vi "Get Measurements P1.vi"(0 "Image In":T1, 11 "Error In":errorcluster) -> (1 "Outer Ring":sgl format="%.2f", 2 "Top Outer":sgl format="%.2f", 3 "Top Inner":sgl format="%.2f", 4 "Image Out":T1, 13 "Number of Matches (Locate P1)":i32, 15 "Error Out":errorcluster)   [LabVIEW 2020]
uses:
  <vilib>/vision/Image Controls.llb/IMAQ Image.ctl
  <vilib>/vision/Pattern Matching.llb/IMAQ Curve Parameters.ctl
  <vilib>/vision/Pattern Matching.llb/IMAQ Match Range Setting.ctl
  <vilib>/vision/Pattern Matching.llb/IMAQ Geometric Pattern 2 Advanced Match Options.ctl
  <vilib>/vision/Image Controls.llb/Vision Info Type2.ctl
  <vilib>/vision/Measure.llb/Edge Options.ctl
  <vilib>/vision/Measure.llb/Edge Polarity.ctl
  <vilib>/vision/NI_Vision_Development_Module.lvlib
panel:
  in  "Template File Path":path=path "C:/Users/serce/Desktop/Smart Vision System Testbench/P1 Pattern.png"
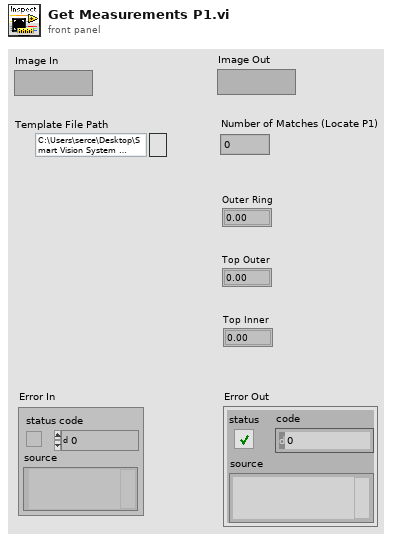
[diagram p1: front panel]
types:
  T1 = typedef "IMAQ Image.ctl" = refnum<image>
  T2 = cluster{"Contrast":i32, "Filter width":i32, "Steepness":i32, "Subsampling Ratio":u32, "Show Search Area":bool, "Show Search Lines":bool, "Show Edges Found":bool, "Show Result":bool}
  T3 = cluster{"Global Rectangle":i32[], "Contours":cluster{"ID":enum32{"External", "Internal"}, "Type":u32, "Coordinates":i32[]}[]}
  T4 = cluster{"Origin":cluster{"X":sgl, "Y":sgl}, "Angle (deg)":sgl, "Axis Reference":u32}
  T5 = enum16{"Reset", "Update Coordinate System", "Get Coordinate System"}
  T6 = typedef "Edge Options.ctl" = cluster{"Edge Polarity":T7, "Kernel Size":u32, "Width":u32, "Minimum Edge Strength":sgl, "Interpolation Type":enum32{"Zero Order", "Bilinear", "Quadratic", "Cubic", "Bilinear Fixed"}, "Data Processing Method":enum32{"Average", "Median"}}
  T7 = typedef "Edge Polarity.ctl" = u32
  T8 = cluster{"Search  Direction":u32, "Edge Options":T6, "Show Search Area":bool, "Show Search Lines":bool, "Show Edges Found":bool, "Show Result":bool, "Search Area Color":u32, "Search Lines Color":u32, "Edge Locations Color":u32, "Result Color":u32, "Overlay Group Name":string}
  T9 = cluster{"Process":enum16{"Get First Edge", "Get First + Last Edge", "Get All Edges", "Get Best Edge"}, "Step Size":i32, "Max Pixel Radius":i32}
  T10 = cluster{"Origin Pixel":cluster{"X":sgl, "Y":sgl}, "Angle Relative to Horizontal (deg)":sgl, "Axis Reference":u32}
  T11 = typedef "Vision Info Type2.ctl" = u32
  T12 = typedef "Simple Grid Descriptor" = cluster{"X Step":sgl, "Y Step":sgl, "Unit":T13}
  T13 = typedef "Image Unit" = enum32{"Undefined", "Angström", "Micrometer", "Millimeter", "Centimeter", "Meter", "Kilometer", "Microinch", "Inch", "Feet", "Nautical miles", "Standard miles", "Steps"}
  T14 = enum16{"Horizontal Motion", "Vertical Motion", "Horizontal and Vertical Motion", "Horizontal, Vertical and Angular Motion"}
  T15 = typedef "IMAQ Curve Parameters.ctl" = cluster{"Extraction Mode":u32, "Edge Threshold":i32, "Edge Filter Size":u32, "Min Length":i32, "Row Search Step Size":i32, "Col Search Step Size":i32, "Max Endpoint Gap":i32, "Closed":bool, "Subpixel":bool}
  T16 = typedef "IMAQ Match Range Setting.ctl" = cluster{"Match Constraints":u32, "Min":dbl, "Max":dbl}
  T17 = typedef "IMAQ Geometric Pattern 2 Advanced Match Options.ctl" = u16
  T18 = cluster{"Curve Parameters":T15, "Match Mode":cluster{"Rotation":bool, "Scale":bool, "Occlusion":bool, "Reserved 1":bool, "Reserved 2":bool, "Reserved 3":bool}, "Range Settings":T16[], "Number of Matches":i32, "Minimum Match Score":sgl, "SubPixel Accuracy":bool, "Adv. Geometric Match Options 2":cluster{"Setup Data Item":T17, "Item Value":dbl}[]}
  T19 = typedef "IMAQ GM Match Report.ctl" = cluster{"Position":cluster{"x":sgl, "y":sgl}, "Angle":sgl, "Scale":sgl, "Score":sgl, "Bounding Box":cluster{"x":sgl, "y":sgl}[], "Contrast Reversed":bool, "Occlusion %":sgl, "Template Target Curve Score":sgl, "Target Template Curve Score":sgl, "Correlation Score":sgl}
  T20 = cluster{"Origin Pixel":cluster{"X":sgl, "Y":sgl}, sgl, "Axis Reference":u32}
  T21 = typedef "IMAQ Coordinate System" = cluster{"Reference System":cluster{"Origin":cluster{"X":sgl, "Y":sgl}, "Angle (deg)":sgl, "Axis Reference":u32}, "Measurement System":cluster{"Origin":cluster{"X":sgl, "Y":sgl}, "Angle (deg)":sgl, "Axis Reference":u32}}
  T22 = typedef "ROI Descriptor" = cluster{"Global Rectangle":i32[], "Contours":cluster{"ID":enum32{"External", "Internal"}, "Type":u32, "Coordinates":i32[]}[]}
  T23 = cluster{"Center (Pixels)":cluster{"X":sgl, "Y":sgl}, "Radius (Pixels)":dbl, "Center (Real-World)":cluster{"X":sgl, "Y":sgl}, "Radius (Real-World)":dbl, "Roundness (Real-World)":dbl, "Average Strength":dbl, "Average SNR (dB)":dbl}
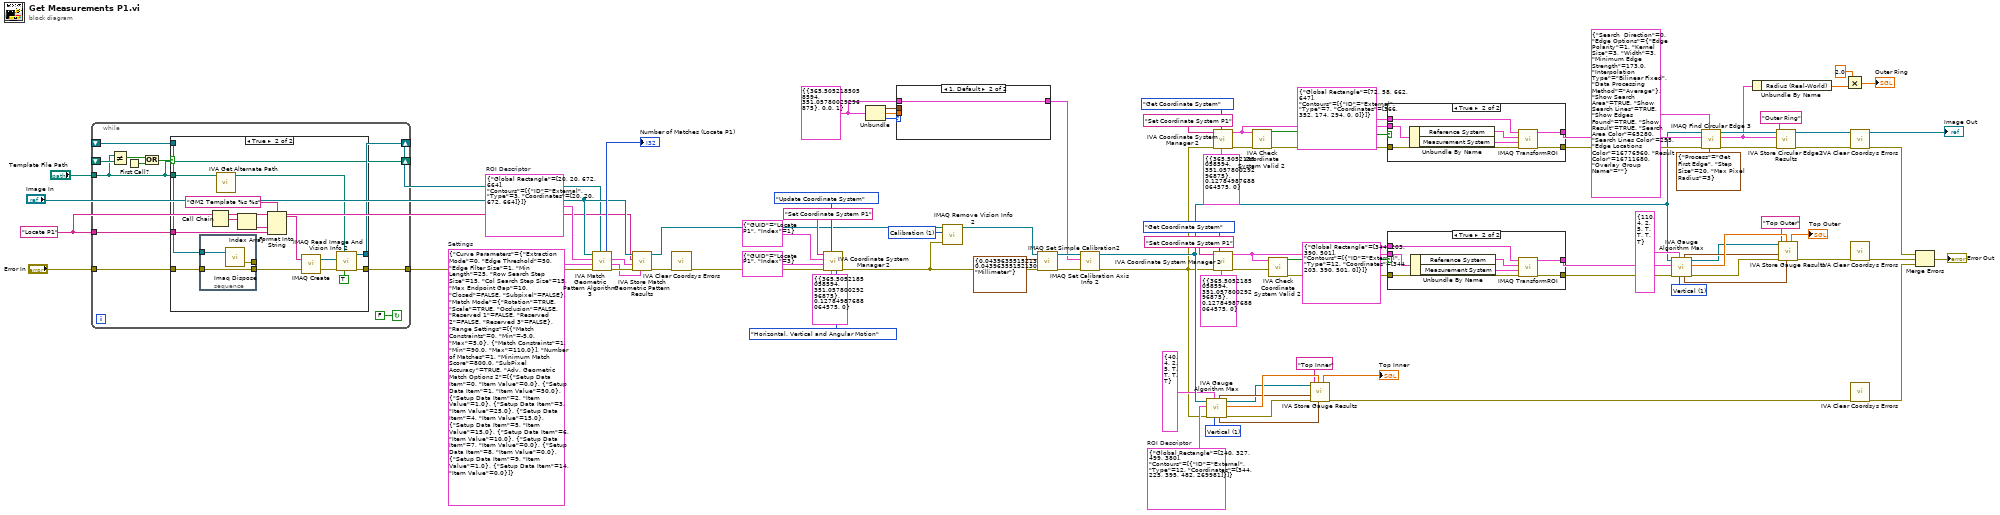
[diagram p0: block diagram]
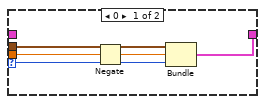
[diagram p4: hidden frame]
diagram:
  w22 = u32 1 items=["Horizontal", "Vertical"] ("Scanning axis")
  w21 = T3 {"Global Rectangle"=[240, 327, 499, 380], "Contours"=[{"ID"=enum."External", "Type"=12, "Coordinates"=[344, 225, 395, 482, 269981]}]}  # ROI Descriptor
  w34 = u32 1 items=["Horizontal", "Vertical"] ("Scanning axis")
  w62 = T10 {"Origin Pixel"={"X"=365.50522, "Y"=351.0578}, "Angle Relative to Horizontal (deg)"=0.0, "Axis Reference"=1} ("Calibration Axis Info")
  w69 = T11 1 items=["Any", "Calibration", "Overlay", "Grayscale Template", "Color Template", "Geometric Template", "Custom Data", "Golden Template", "Geometric Template 2", "Contour Data", "Camera Model"] ("Vision Info")
  w82 = T18 {"Curve Parameters"={"Extraction Mode"=0, "Edge Threshold"=50, "Edge Filter Size"=1, "Min Length"=25, "Row Search Step Size"=15, "Col Search Step Size"=15, "Max Endpoint Gap"=10, "Closed"=FALSE, "Subpixel"=FALSE}, "Match Mode"={"Rotation"=TRUE, "Scale"=TRUE, "Occlusion"=FALSE, "Reserved 1"=FALSE, "Reserved 2"=FALSE, "Reserved 3"=FALSE}, "Range Settings"=[{"Match Constraints"=0, "Min"=-5.0, "Max"=5.0}, {"Match Constraints"=1, "Min"=90.0, "Max"=110.0}], "Number of Matches"=1, "Minimum Match Score"=800.0, "SubPixel Accuracy"=TRUE, "Adv. Geometric Match Options 2"=[{"Setup Data Item"=0, "Item Value"=0.0}, {"Setup Data Item"=1, "Item Value"=50.0}, {"Setup Data Item"=2, "Item Value"=1.0}, {"Setup Data Item"=3, "Item Value"=25.0}, {"Setup Data Item"=4, "Item Value"=15.0}, {"Setup Data Item"=5, "Item Value"=15.0}, {"Setup Data Item"=6, "Item Value"=10.0}, {"Setup Data Item"=7, "Item Value"=0.0}, {"Setup Data Item"=8, "Item Value"=0.0}, {"Setup Data Item"=9, "Item Value"=1.0}, {"Setup Data Item"=14, "Item Value"=0.0}]}  # Settings
  w81 = "Locate P1" ("Step Name")
  w89 = T3 {"Global Rectangle"=[20, 20, 672, 664], "Contours"=[{"ID"=enum."External", "Type"=3, "Coordinates"=[20, 20, 672, 664]}]}  # ROI Descriptor
  n1 = while {
    shift-right: [w101] -> w79
    shift-left: _ -> [w100]
    tunnel: [w98] -> w80
    tunnel: "Error In" -> [w97]
    tunnel: "Template File Path" -> [w94]
    tunnel: w81 -> [w96]
    shift-right: [w94] -> _
    shift-left: _ -> [w95]
    stop <- FALSE continue-if-true
    n2 = Not Equal?(x=w94, y=w95) -> (x != y?=w92:bool)
    n3 = First Call?() -> (First Call?: T/F=w93:bool)
    n4 = Or(x=w92, y=w93) -> (x .or. y?=w91:bool)
    n5 = case shown="True" w91 {
      tunnel: [w103 w105] -> w101
      tunnel: w100 -> [w103 w112]
      tunnel: [w102 w107] -> w98
      tunnel: w97 -> [w102 w113]
      tunnel: w96 -> [_ w114]
      tunnel: w94 -> [_ w111]
      frame False {
      }
      frame True {
        n6 = stacked-sequence {
          tunnel: w113 -> [w121]
          tunnel: w112 -> [w120]
          tunnel: [w121] -> w110
          tunnel: [w119] -> _
          frame #0 {
            n7 = call "Imaq Dispose"("Image"=w120) -> ("error out"=w119:errorcluster)  [unwired: 2 in, 3 out]
          }
        }
        n8 = Call Chain() -> (call chain=w116:string[])
        n9 = call <vilib>:"IVA Get Alternate Path.vi"("Path In"=w111) -> ("Path Out"=w106:path)  [unwired: 10 out]
        n10 = Index Array(array=w116) -> (element=w115:string)  [unwired: 1 in]
        n11 = Format Into String(format string="GM2 Template %s %s" ("Image Name"), w115, w114) -> (resulting string=w118:string)  [unwired: 2 in, 1 out]
        n12 = call "IMAQ Create"("Image Name"=w118, "error in (no error)"=w110) -> ("New Image"=w104:T1, "error out"=w108:errorcluster)  [unwired: 2 in, 1 out]
        n13 = call "IMAQ Read Image And Vision Info 2"("Use File Path Image Type"=TRUE, "File Path"=w106, "error in (no error)"=w108, "Image"=w104) -> ("error out"=w107:errorcluster, "Image Out"=w105:T1)  [unwired: 5 in, 1 out]
      }
    }
  }
  n14 = call <vilib>:"IVA Match Geometric Pattern Algorithm 3.vi"("Template"=w79, "error in (no error)"=w80, "Settings"=w82, "ROI Descriptor"=w89, "Image"="Image In") -> ("error out"=w88:errorcluster, "Calibrated Matches"=w86:T19[], "Matches"=w87:T19[], "Number of Matches"=→"Number of Matches (Locate P1)":i32)  [unwired: 3 out]
  n15 = call <vilib>:"IVA Store Match Geometric Pattern Results.vi"("Calibrated Matches"=w86, "error in (no error)"=w88, "Matches"=w87, "Step Name"=w81, "Image in"="Image In") -> ("error out"=w78:errorcluster, "Image dup"=w68:T1)  [unwired: 5 out]
  n16 = call <vilib>:"IVA Clear Coordsys Errors.vi"("error in (no error)"=w78) -> ("error out"=w71:errorcluster)  [unwired: 10 in]
  n17 = call <vilib>:"IVA Coordinate System Manager 2.vi"("Mode"=T14."Horizontal, Vertical and Angular Motion", "Reference System"=T4 {"Origin"={"X"=365.50522, "Y"=351.0578}, "Angle (deg)"=0.12784988, "Axis Reference"=0}, "Function"=T5."Update Coordinate System", "error in (no error)"=w71, "Angle ID"=cluster{"GUID":string, "Index":i32} {"GUID"="Locate P1", "Index"=3}, "Origin ID"=cluster{"GUID":string, "Index":i32} {"GUID"="Locate P1", "Index"=1}, "Coordinate System Name"="Set Coordinate System P1") -> ("error out"=w66:errorcluster)  [unwired: 4 out]
  n18 = Unbundle(w62) -> ("Origin Pixel"=w59:cluster{"X":sgl, "Y":sgl}, "Angle Relative to Horizontal (deg)"=w60:sgl, "Axis Reference"=w63:u32)
  n19 = case shown="1, Default" w63 {
    selector: w63 -> [w123 _]
    tunnel: w62 -> [_ w127]
    tunnel: [w122 w127] -> w61
    tunnel: w60 -> [w126 _]
    tunnel: w59 -> [w125 _]
    frame 0 {
      n20 = Negate(x=w126) -> (-x=w124:sgl)
      n21 = Bundle("Origin Pixel"=w125, w124, "Axis Reference"=w123) -> (w122:T20)  [unwired: 1 in]
    }
    frame 1, Default {
    }
  }
  n22 = call "IMAQ Remove Vision Info 2"("error in (no error)"=w66, "Vision Info"=w69, "Image"=w68) -> ("Image Out"=w67:T1)  [unwired: 8 out]
  n23 = call "IMAQ Set Simple Calibration2"("error in (no error)"=w66, "Pixel Distances"=T12 {"X Step"=0.04396355, "Y Step"=0.04396355, "Unit"=enum."Millimeter"} ("Grid Descriptor"), "Image"=w67) -> ("error out"=w64:errorcluster, "Calibration Template Image"=w65:T1)  [unwired: 2 in, 5 out]
  n24 = call-poly "IMAQ Set Calibration Axis Info 2"("error in (no error)"=w64, "Calibration Axis Info"=w61, "Calibration Template Image In"=w65) -> ("error out"=w17:errorcluster, "Calibration Template Image Out"=w24:T1)  [unwired: 7 out]
  n25 = call <vilib>:"IVA Gauge Algorithm Max.vi"("Scanning axis"=w22, "Settings"=T2 {"Contrast"=40, "Filter width"=4, "Steepness"=2, "Subsampling Ratio"=5, "Show Search Area"=TRUE, "Show Search Lines"=TRUE, "Show Edges Found"=TRUE, "Show Result"=TRUE}, "error in (no error)"=w17, "ROI Descriptor"=w21, "Image"=w24) -> ("error out"=w13:errorcluster, "Distance"=w20:sgl, "Image Out"=w14:T1, "Distance Points"=w12:cluster{"X":sgl, "Y":sgl}[], "Points of Contact"=w19:cluster{"X":sgl, "Y":sgl}[])  [unwired: 1 in, 1 out]
  n26 = call <vilib>:"IVA Coordinate System Manager 2.vi"("Reference System"=T4 {"Origin"={"X"=365.50522, "Y"=351.0578}, "Angle (deg)"=0.12784988, "Axis Reference"=0}, "Function"=T5."Get Coordinate System", "error in (no error)"=w17, "Coordinate System Name"="Set Coordinate System P1") -> ("error out"=w52:errorcluster, "Coordinate System Out"=w54:T21)  [unwired: 3 in, 3 out]
  n27 = call <vilib>:"IVA Coordinate System Manager 2.vi"("Reference System"=T4 {"Origin"={"X"=365.50522, "Y"=351.0578}, "Angle (deg)"=0.12784988, "Axis Reference"=0}, "Function"=T5."Get Coordinate System", "error in (no error)"=w17, "Coordinate System Name"="Set Coordinate System P1") -> ("error out"=w37:errorcluster, "Coordinate System Out"=w39:T21)  [unwired: 3 in, 3 out]
  n28 = call <vilib>:"IVA Check Coordinate System Valid 2.vi"("error in (no error)"=w52, "Coordinate System"=w54) -> ("error out"=w51:errorcluster, "Valid?"=w53:bool)  [unwired: 8 out]
  n29 = call <vilib>:"IVA Check Coordinate System Valid 2.vi"("error in (no error)"=w37, "Coordinate System"=w39) -> ("error out"=w36:errorcluster, "Valid?"=w38:bool)  [unwired: 8 out]
  n30 = call <vilib>:"IVA Store Gauge Results.vi"("Distance Points"=w12, "Distance"=w20, "error in (no error)"=w13, "Points of Contact"=w19, "Step Name"="Top Inner", "Image in"=w14) -> ("error out"=w15:errorcluster, "Distance (calibrated)"=→"Top Inner":sgl)  [unwired: 4 out]
  n31 = case shown="True" w53 {
    tunnel: T3 {"Global Rectangle"=[72, 58, 662, 647], "Contours"=[{"ID"=enum."External", "Type"=7, "Coordinates"=[366, 352, 174, 294, 0, 0]}]} ("ROI Descriptor") -> [w129 w136]
    tunnel: [w129 w135] -> w49
    tunnel: [w128 w134] -> w48
    tunnel: w54 -> [_ w133]
    tunnel: w51 -> [w128 w132]
    frame False {
    }
    frame True {
      n32 = Unbundle By Name(w133) -> ("Reference System"=w131:T4, "Measurement System"=w130:T4)
      n33 = call "IMAQ TransformROI"("error in (no error)"=w132, "New Reference"=w130, "Base Reference"=w131, "ROI Descriptor"=w136) -> ("error out"=w134:errorcluster, "ROI Descriptor out"=w135:T22)  [unwired: 6 out]
    }
  }
  n34 = case shown="True" w38 {
    tunnel: T3 {"Global Rectangle"=[344, 203, 390, 501], "Contours"=[{"ID"=enum."External", "Type"=12, "Coordinates"=[344, 203, 390, 501, 0]}]} ("ROI Descriptor") -> [w138 w145]
    tunnel: [w138 w142] -> w2
    tunnel: [w137 w141] -> w30
    tunnel: w39 -> [_ w140]
    tunnel: w36 -> [w137 w139]
    frame False {
    }
    frame True {
      n35 = Unbundle By Name(w140) -> ("Reference System"=w144:T4, "Measurement System"=w143:T4)
      n36 = call "IMAQ TransformROI"("error in (no error)"=w139, "New Reference"=w143, "Base Reference"=w144, "ROI Descriptor"=w145) -> ("error out"=w141:errorcluster, "ROI Descriptor out"=w142:T22)  [unwired: 6 out]
    }
  }
  n37 = call <vilib>:"IVA Gauge Algorithm Max.vi"("Scanning axis"=w34, "Settings"=T2 {"Contrast"=110, "Filter width"=4, "Steepness"=2, "Subsampling Ratio"=5, "Show Search Area"=TRUE, "Show Search Lines"=TRUE, "Show Edges Found"=TRUE, "Show Result"=TRUE}, "error in (no error)"=w30, "ROI Descriptor"=w2, "Image"=w24) -> ("error out"=w26:errorcluster, "Distance"=w33:sgl, "Image Out"=w27:T1, "Distance Points"=w25:cluster{"X":sgl, "Y":sgl}[], "Points of Contact"=w32:cluster{"X":sgl, "Y":sgl}[])  [unwired: 1 in, 1 out]
  n38 = call "IMAQ Find Circular Edge 3"("Circle Fit Options"=T9 {"Process"=enum."Get First Edge", "Step Size"=20, "Max Pixel Radius"=3}, "Options"=T8 {"Search  Direction"=0, "Edge Options"={"Edge Polarity"=1, "Kernel Size"=3, "Width"=3, "Minimum Edge Strength"=173.0, "Interpolation Type"=enum."Bilinear Fixed", "Data Processing Method"=enum."Average"}, "Show Search Area"=TRUE, "Show Search Lines"=TRUE, "Show Edges Found"=TRUE, "Show Result"=TRUE, "Search Area Color"=65280, "Search Lines Color"=255, "Edge Locations Color"=16776960, "Result Color"=16711680, "Overlay Group Name"=""}, "error in (no error)"=w48, "ROI Descriptor"=w49, "Image"=w24) -> ("error out"=w45:errorcluster, "Fitted Circle"=w5:T23, "Image Out"=w44:T1)  [unwired: 2 in, 2 out]
  n39 = Unbundle By Name(w5) -> ("Radius (Real-World)"=w7:dbl)
  n40 = call <vilib>:"IVA Store Circular Edge2 Results.vi"("error in (no error)"=w45, "Step Name"="Outer Ring", "Fitted Circle"=w5, "Image in"=w44) -> ("error out"=w43:errorcluster, "Image dup"=→"Image Out":T1)  [unwired: 2 in, 4 out]
  n41 = call <vilib>:"IVA Store Gauge Results.vi"("Distance Points"=w25, "Distance"=w33, "error in (no error)"=w26, "Points of Contact"=w32, "Step Name"="Top Outer", "Image in"=w27) -> ("error out"=w28:errorcluster, "Distance (calibrated)"=→"Top Outer":sgl)  [unwired: 4 out]
  n42 = Multiply(x=2.0, y=w7) -> (x*y=→"Outer Ring":dbl)
  n43 = call <vilib>:"IVA Clear Coordsys Errors.vi"("error in (no error)"=w43) -> ("error out"=w10:errorcluster)  [unwired: 10 in]
  n44 = call <vilib>:"IVA Clear Coordsys Errors.vi"("error in (no error)"=w28) -> ("error out"=w9:errorcluster)  [unwired: 10 in]
  n45 = call <vilib>:"IVA Clear Coordsys Errors.vi"("error in (no error)"=w15) -> ("error out"=w8:errorcluster)  [unwired: 10 in]
  n46 = Merge Errors(w10, w9, w8) -> (→"Error Out":errorcluster)
